vi "flyback_tri.vi"(6 "mode":u16(ring) items=["step", "line", "3-rd", "sine"], 8 "points in t1":dbl=500.0, 9 "points in t2":dbl=500.0, 10 "p2":dbl=10000.0, 11 "p1":dbl=10000.0) -> (3 "array":dbl[](array[numeric]))   [LabVIEW 2015]
uses:
  <vilib>/Analysis/7linalg.llb/Solve Linear Equations (single right hand).vi
  <vilib>/Analysis/baseanly.llb/Solve Linear Equations By Cholesky.vi
  <vilib>/Analysis/baseanly.llb/Real Matrix to Compact Array.vi
  <vilib>/Analysis/baseanly.llb/Real Compact Tri-Matrix Linear Eqs.vi
  <vilib>/Analysis/7linalg.llb/Solve Linear Eqs (General).vi
  <vilib>/Analysis/7linalg.llb/Solve Linear Eqs (Gen, single right hand).vi
  <vilib>/Analysis/NI_AALPro.lvlib
panel:
  out "deleted portion 2":dbl
  out "deleted portion":dbl
  out "x":dbl[](array[numeric])
  out "B":dbl[](array[numeric])
  out "A":dbl[][](array[numeric])
  out "Waveform Graph":dbl[](graph)
  out "b":dbl=10000.0
  out "a":dbl=10000.0
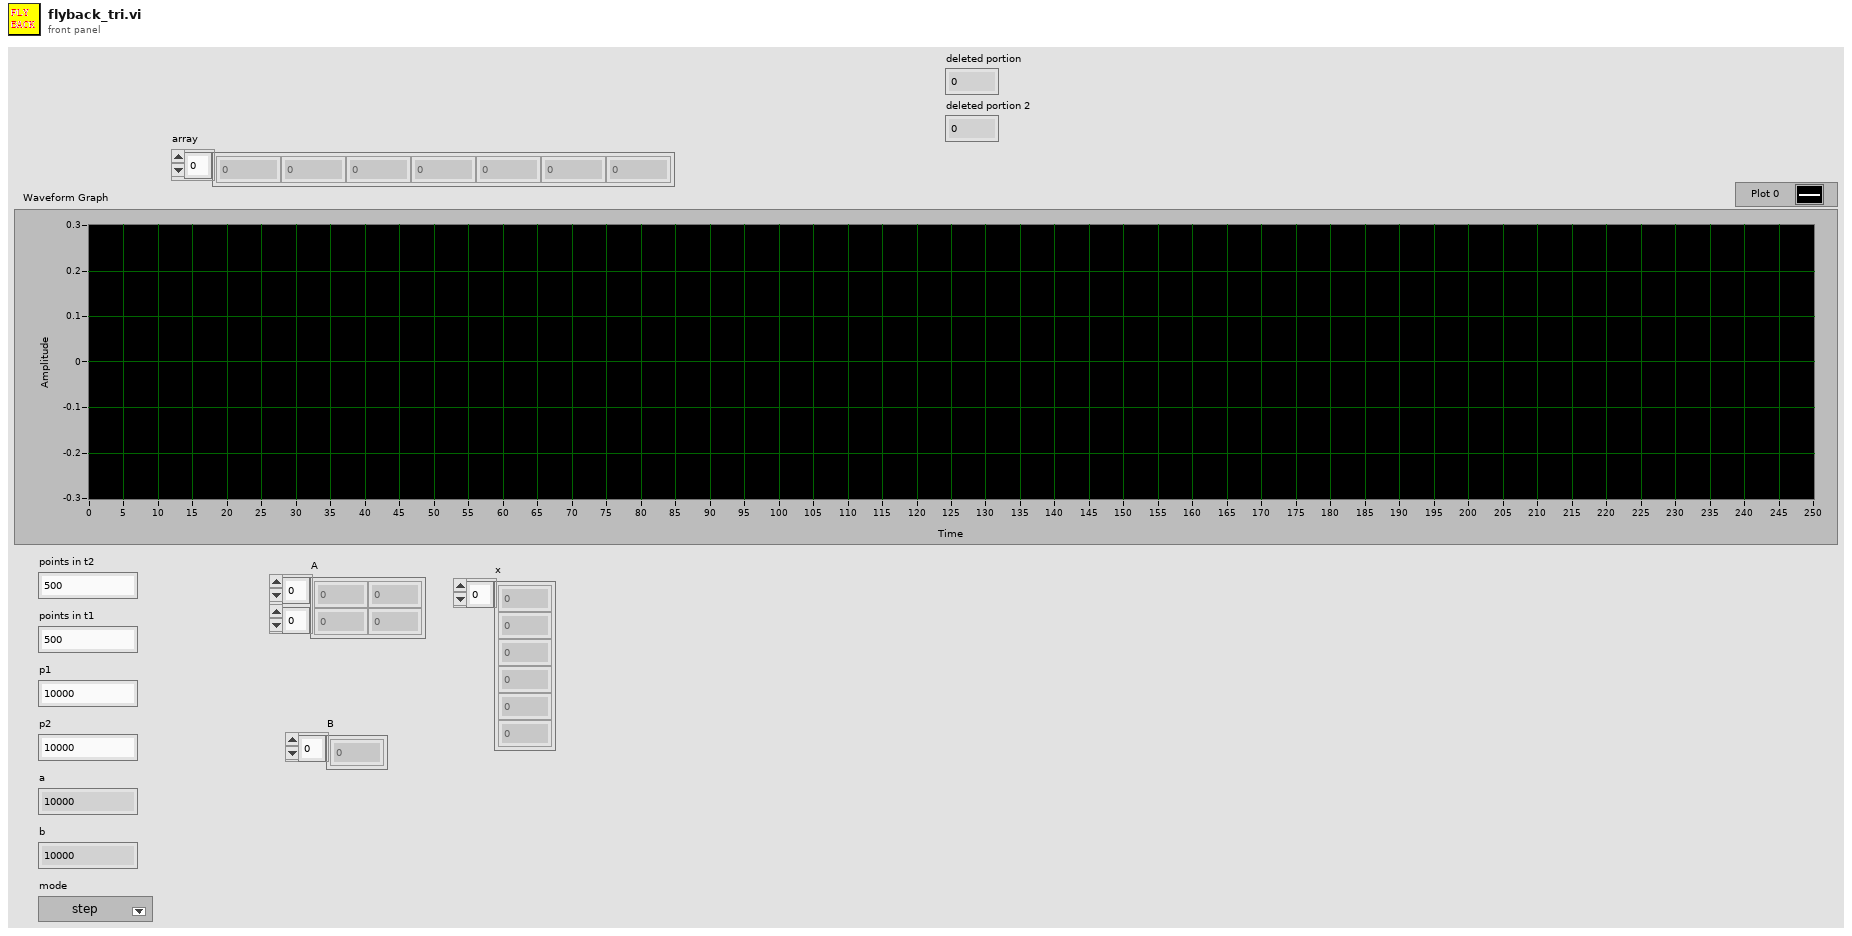
[diagram p1: front panel]
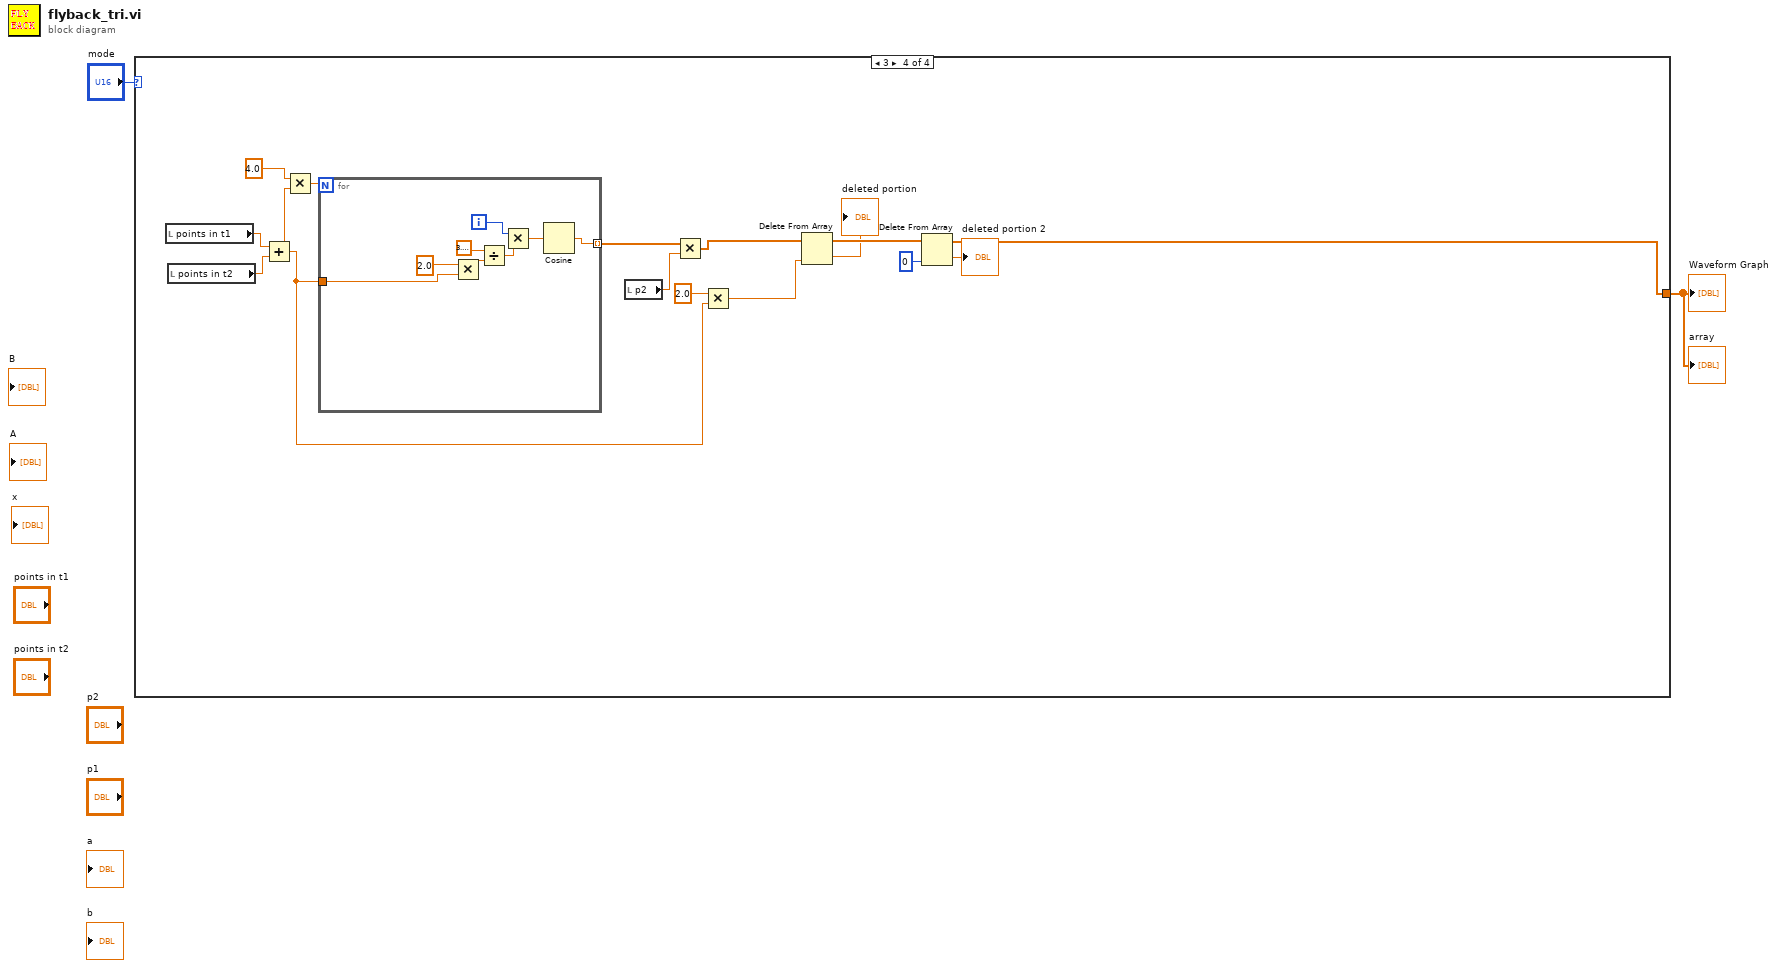
[diagram p0: block diagram]
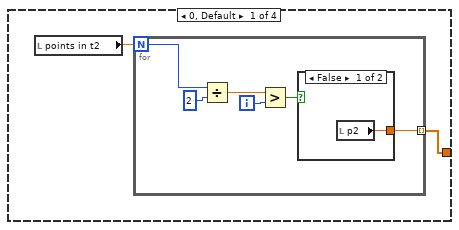
[diagram p2: hidden frame]
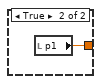
[diagram p3: hidden frame]
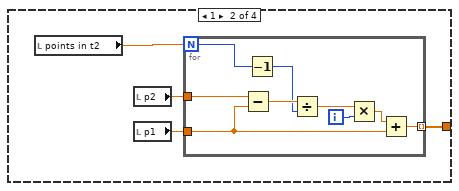
[diagram p4: hidden frame]
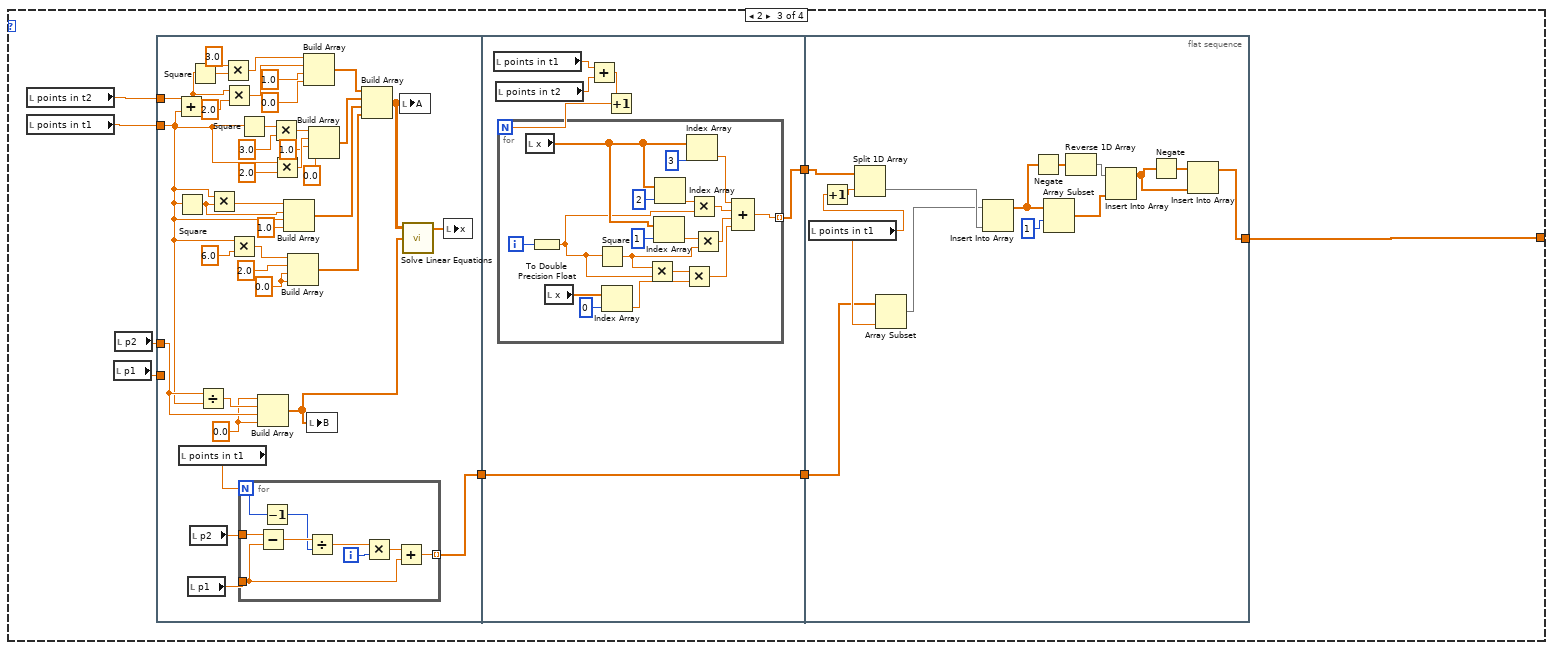
[diagram p5: hidden frame]
diagram:
  n1 = case shown="3" "mode" {
    tunnel: [w4 w16 w26 w121] -> w1
    frame 0, Default {
      n2 = local read "points in t2"() -> (w3:dbl)
      n3 = for {
        N: w3 -> [w9]
        tunnel: [w5] -> w4 mode=indexing
        i -> [w7]
        n4 = Divide(x=w9, y=2) -> (x/y=w8:dbl)
        n5 = Greater?(x=w8, y=w7) -> (0:w6:bool)
        n6 = case shown="False" w6 {
          tunnel: [w11 w12] -> w5
          frame False {
            n7 = local read "p2"() -> (w11:dbl)
          }
          frame True {
            n8 = local read "p1"() -> (w12:dbl)
          }
        }
      }
    }
    frame 1 {
      n9 = local read "points in t2"() -> (w14:dbl)
      n10 = local read "p2"() -> (w15:dbl)
      n11 = local read "p1"() -> (w13:dbl)
      n12 = for {
        N: w14 -> [w23]
        tunnel: w15 -> [w25]
        tunnel: w13 -> [w19]
        tunnel: [w17] -> w16 mode=indexing
        i -> [w21]
        n13 = Subtract(x=w25, y=w19) -> (x-y=w24:dbl)
        n14 = Decrement(x=w23) -> (x-1=w22:i32)
        n15 = Divide(x=w24, y=w22) -> (x/y=w20:dbl)
        n16 = Multiply(x=w20, y=w21) -> (x*y=w18:dbl)
        n17 = Add(x=w18, y=w19) -> (x+y=w17:dbl)
      }
    }
    frame 2 {
      n18 = local read "points in t2"() -> (w28:dbl)
      n19 = local read "points in t1"() -> (w27:dbl)
      n20 = local read "p1"() -> (w33:dbl)
      n21 = local read "p2"() -> (w32:dbl)
      n22 = flat-sequence {
        tunnel: w28 -> [w60]
        tunnel: w32 -> [w42]
        tunnel: w33 -> [_]
        tunnel: w27 -> [w38]
        tunnel: [w68] -> w29
        tunnel: [w86] -> w31
        tunnel: [w85] -> w30
        tunnel: w29 -> [w85]
        tunnel: w31 -> [w110]
        tunnel: w30 -> [w115]
        tunnel: [w105] -> w26
        frame #0 {
          w34 = 0.0 ("element")
          w36 = 0.0 ("element")
          n23 = Add(x=w60, y=w38) -> (x+y=w56:dbl)
          n24 = Square(x=w38) -> (x^2=w50:dbl)
          n25 = local read "points in t1"() -> (w71:dbl)
          n26 = local read "p1"() -> (w69:dbl)
          n27 = Square(x=w56) -> (x^2=w59:dbl)
          n28 = local read "p2"() -> (w70:dbl)
          n29 = Divide(x=w42, y=w38) -> (x/y=w35:dbl)
          n30 = Multiply(x=w38, y=w50) -> (x*y=w51:dbl)
          n31 = Multiply(x=3.0, y=w59) -> (x*y=w57:dbl)
          n32 = Multiply(x=w56, y=2.0) -> (x*y=w54:dbl)
          n33 = Multiply(x=w38, y=6.0) -> (x*y=w44:dbl)
          n34 = Square(x=w38) -> (x^2=w67:dbl)
          n35 = for {
            N: w71 -> [w78]
            tunnel: w70 -> [w80]
            tunnel: w69 -> [w74]
            tunnel: [w72] -> w68 mode=indexing
            i -> [w76]
            n36 = Subtract(x=w80, y=w74) -> (x-y=w79:dbl)
            n37 = Decrement(x=w78) -> (x-1=w77:i32)
            n38 = Divide(x=w79, y=w77) -> (x/y=w75:dbl)
            n39 = Multiply(x=w75, y=w76) -> (x*y=w73:dbl)
            n40 = Add(x=w73, y=w74) -> (x+y=w72:dbl)
          }
          n41 = Build Array(w34, w35, w42, w34) -> (w40:dbl[])
          n42 = Multiply(x=w67, y=3.0) -> (x*y=w65:dbl)
          n43 = Multiply(x=w38, y=2.0) -> (x*y=w63:dbl)
          n44 = Build Array(w51, w50, w38, 1.0 ("element")) -> (w46:dbl[])
          n45 = Build Array(w44, 2.0 ("y"), w36, w36) -> (w43:dbl[])
          n46 = Build Array(w57, w54, 1.0, 0.0 ("element")) -> (w48:dbl[])
          n47 = local write "B"(w40) -> ()
          n48 = Build Array(w65, w63, 1.0 ("element"), 0.0 ("element")) -> (w47:dbl[])
          n49 = Build Array(w48, w47, w46, w43) -> (w39:dbl[][])
          n50 = local write "A"(w39) -> ()
          n51 = call-poly <vilib>:"Solve Linear Equations.vi"("Known Vector"=w40, "Input Matrix"=w39) -> ("Solution Vector"=w41:dbl[])  [unwired: 1 in, 1 out]
          n52 = local write "x"(w41) -> ()
        }
        frame #1 {
          n53 = local read "points in t1"() -> (w84:dbl)
          n54 = local read "points in t2"() -> (w83:dbl)
          n55 = Add(x=w84, y=w83) -> (x+y=w82:dbl)
          n56 = Increment(x=w82) -> (x+1=w81:dbl)
          n57 = for {
            N: w81 -> [_]
            tunnel: [w104] -> w86 mode=indexing
            i -> [w103]
            n58 = local read "x"() -> (w96:dbl[])
            n59 = To Double Precision Float(number=w103) -> (double precision float=w91:dbl)
            n60 = local read "x"() -> (w90:dbl[])
            n61 = Square(x=w91) -> (x^2=w92:dbl)
            n62 = Index Array(array=w90, index=0) -> (element=w88:dbl)
            n63 = Multiply(x=w92, y=w91) -> (x*y=w89:dbl)
            n64 = Index Array(array=w96, index=1) -> (element=w95:dbl)
            n65 = Index Array(array=w96, index=2) -> (element=w98:dbl)
            n66 = Multiply(x=w89, y=w88) -> (x*y=w87:dbl)
            n67 = Index Array(array=w96, index=3) -> (element=w101:dbl)
            n68 = Multiply(x=w98, y=w91) -> (x*y=w100:dbl)
            n69 = Multiply(x=w95, y=w92) -> (x*y=w94:dbl)
            n70 = Compound Arithmetic op=ADD(w101, w100, w94, w87) -> (w104:dbl)
          }
        }
        frame #2 {
          n71 = local read "points in t1"() -> (w118:dbl)
          n72 = Increment(x=w118) -> (x+1=w107:dbl)
          n73 = Split 1D Array(array=w110, index=w107) -> (second subarray=w109:dbl[])  [unwired: 1 out]
          n74 = Array Subset(array=w115, length=w118) -> (w108:dbl[])  [unwired: 1 in]
          n75 = Insert Into Array(array=w108, new element=w109) -> (w106:dbl[])  [unwired: 1 in]
          n76 = Negate(x=w106) -> (-x=w116:dbl[])
          n77 = Array Subset(array=w106, index=1) -> (w113:dbl[])  [unwired: 1 in]
          n78 = Reverse 1D Array(array=w116) -> (reversed array=w117:dbl[])
          n79 = Insert Into Array(array=w117, new element=w113) -> (w111:dbl[])  [unwired: 1 in]
          n80 = Negate(x=w111) -> (-x=w112:dbl[])
          n81 = Insert Into Array(array=w112, new element=w111) -> (w105:dbl[])  [unwired: 1 in]
        }
      }
    }
    frame 3 {
      n82 = local read "points in t1"() -> (w130:dbl)
      n83 = local read "points in t2"() -> (w131:dbl)
      n84 = Add(x=w130, y=w131) -> (x+y=w126:dbl)
      n85 = Multiply(x=4.0, y=w126) -> (x*y=w129:dbl)
      n86 = for {
        N: w129 -> [_]
        tunnel: [w140] -> w133 mode=indexing
        tunnel: w126 -> [w134]
        i -> [w139]
        n87 = Multiply(x=2.0, y=w134) -> (x*y=w136:dbl)
        n88 = Divide(x=3.141592653589793, y=w136) -> (x/y=w138:dbl)
        n89 = Multiply(x=w139, y=w138) -> (x*y=w141:dbl)
        n90 = Cosine(x=w141) -> (cos(x)=w140:dbl)
      }
      n91 = local read "p2"() -> (w132:dbl)
      n92 = Multiply(x=w133, y=w132) -> (x*y=w127:dbl[])
      n93 = Multiply(x=2.0, y=w126) -> (x*y=w124:dbl)
      n94 = Delete From Array(array=w127, index=w124) -> (deleted portion=→"deleted portion":dbl, array with subset deleted=w123:dbl[])  [unwired: 1 in]
      n95 = Delete From Array(array=w123, index=0) -> (deleted portion=→"deleted portion 2":dbl, array with subset deleted=w121:dbl[])  [unwired: 1 in]
    }
  }
  "array" <- w1
  "Waveform Graph" <- w1
